vi "7HP_Channels.vi"(1 "Analysis Info cluster":T2[](array[typedef]) {"Sync Delay Time (s)" format="%.4f"; "Sd Error in Variance" format="%.2f"; "Skew_u" format="%.2f"; "% u'/U" format="%.2f"; "Sd Error in Mean" format="%.2f"; "Kurt_u" format="%.2f"; "u^4" format="%.2f"; "u^3" format="%.2f"; "U" format="%.2f"; "u^2" format="%.2f"}) -> (0 "7HP Info":T1(array[cluster]))   [LabVIEW 2017]
uses:
  Controls/Analysis_info_cluster.ctl
  Controls/Inst_type.ctl
  Controls/Instrument_Array.ctl
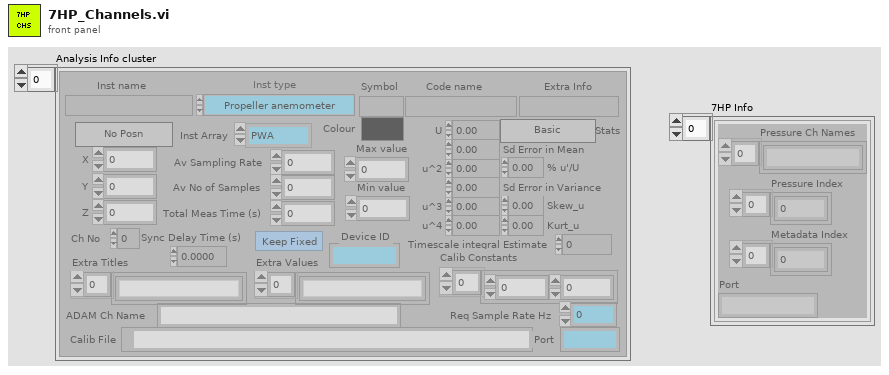
[diagram p1: front panel]
types:
  T1 = cluster{"Pressure Ch Names":string[], "Pressure Index":i32[], "Metadata Index":i32[], "Port":string}[]
  T2 = typedef "Analysis_info_cluster.ctl" = cluster{"Colour":u32, "Inst type":T3, "Inst name":string, "Symbol":string, "Code name":string, "Extra Info":string, "Inst Array":T4, "Extra Titles":string[], "Extra Values":string[], "U":dbl, "u^2":dbl, "u^3":dbl, "u^4":dbl, "Skew_u":dbl, "Kurt_u":dbl, "Sd Error in Mean":dbl, "% u'/U":dbl, "X":dbl, "Y":dbl, "Z":dbl, "Timescale integral Estimate":dbl, "Sd Error in Variance":dbl, "Calib File":path, "Calib Constants":dbl[], "Output Position":bool, "Full Stats":bool, "Av Sampling Rate":dbl, "Av No of Samples":dbl, "Total Meas Time (s)":dbl, "ADAM Ch Name":string, "Max value":dbl, "Min value":dbl, "Req Sample Rate Hz":dbl, "Sync Delay Time (s)":dbl, "Ch No":i16, "Device ID":string, "Use Latest Calib":bool, "Port":string}
  T3 = typedef "Inst_type.ctl" = enum16{"Propeller anemometer", "Raw voltage", "Pressure Transducer", "Pitot-static tube", "Preston tube", "Hot wire", "Cross wire 1", "Cross wire 2", "Generic Linear", "Generic Polynomial", "Generic BackPoly", "Fast FID", "Thermocouple", "Cold wire", "Pulsed Wire", "LDA Vel", "LDA Tran time", "LDA Arr time", "Microphone"}
  T4 = typedef "Instrument_Array.ctl" = enum16{"PWA", "LDA", "Analogue"}
  T5 = cluster{"Pressure Ch Names":string[], "Pressure Index":i32[], "Metadata Index":i32[], "Port":string}
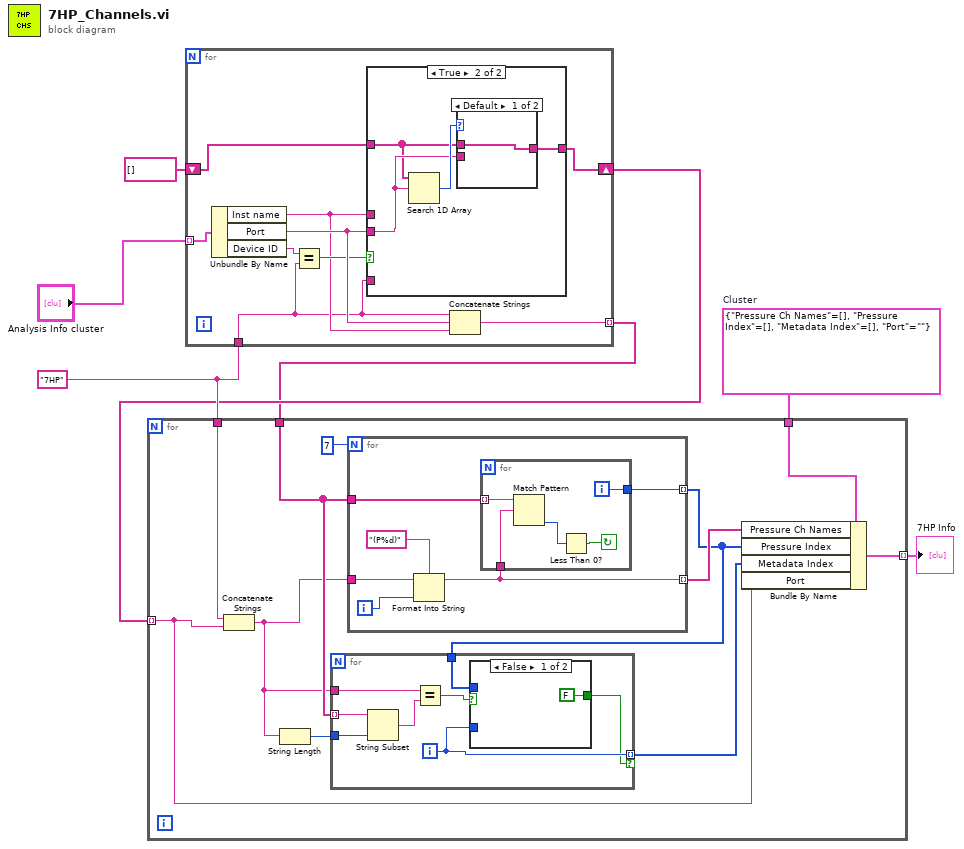
[diagram p0: block diagram]
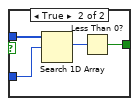
[diagram p2: hidden frame]
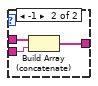
[diagram p4: hidden frame]
diagram:
  w2 = T5 {"Pressure Ch Names"=[], "Pressure Index"=[], "Metadata Index"=[], "Port"=""}  # Cluster
  w5 = "7HP" ("Device ID")
  n1 = for {
    tunnel: "Analysis Info cluster" -> [w11] mode=indexing
    shift-right: [w13] -> w4
    shift-left: string[] [] -> [w15]
    tunnel: [w9] -> w3 mode=indexing
    tunnel: w5 -> [w8]
    n2 = Unbundle By Name(w11) -> ("Inst name"=w10:string, "Port"=w14:string, "Device ID"=w16:string)
    n3 = Equal?(x=w16, y=w8) -> (x = y?=w12:bool)
    n4 = case shown="True" w12 {
      tunnel: w15 -> [w17 w18]
      tunnel: w14 -> [_ w19]
      tunnel: [w17 w20] -> w13
      tunnel: w8 -> [_ _]
      tunnel: w10 -> [_ _]
      frame False {
      }
      frame True {
        n5 = Search 1D Array(1D array=w18, element=w19) -> (index of element=w21:i32)  [unwired: 1 in]
        n6 = case shown="Default" w21 {
          tunnel: w18 -> [w22 w25]
          tunnel: w19 -> [_ w24]
          tunnel: [w22 w23] -> w20
          frame Default {
          }
          frame -1 {
            n7 = Build Array (concatenate)(w25, w24) -> (w23:string[])
          }
        }
      }
    }
    n8 = Concatenate Strings(w8, w14, w10) -> (w9:string)
  }
  n9 = for {
    tunnel: w5 -> [w36]
    tunnel: w4 -> [w32] mode=indexing
    tunnel: w3 -> [w30]
    tunnel: w2 -> [w34]
    tunnel: [w26] -> w1 mode=indexing
    n10 = Concatenate Strings(w36, w32) -> (w29:string)
    n11 = String Length(string=w29) -> (length=w31:i32)
    n12 = for {
      N: 7 -> [_]
      tunnel: w30 -> [w53]
      tunnel: [w52] -> w28 mode=indexing
      tunnel: w29 -> [w51]
      tunnel: [w50] -> w33 mode=indexing
      i -> [w55]
      n13 = Format Into String(format string="(P%d)", initial string=w51, w55) -> (resulting string=w50:string)  [unwired: 1 in, 1 out]
      n14 = for {
        tunnel: w53 -> [w56] mode=indexing
        tunnel: w50 -> [w60]
        tunnel: [w57] -> w52
        i -> [w57]
        stop <- w59 continue-if-true
        n15 = Match Pattern(string=w56, regular expression=w60) -> (offset past match=w58:i32)  [unwired: 1 in, 3 out]
        n16 = Less Than 0?(x=w58) -> (x < 0?=w59:bool)
      }
    }
    n17 = for {
      tunnel: w31 -> [w44]
      tunnel: w30 -> [w43] mode=indexing
      tunnel: w29 -> [w41]
      tunnel: w28 -> [w39]
      tunnel: [w38] -> w27 mode=indexing if=w37
      i -> [w38]
      n18 = String Subset(string=w43, length (rest)=w44) -> (substring=w42:string)  [unwired: 1 in]
      n19 = Equal?(x=w41, y=w42) -> (x = y?=w40:bool)
      n20 = case shown="False" w40 {
        tunnel: w39 -> [_ w49]
        tunnel: w38 -> [_ w48]
        tunnel: [FALSE w46] -> w37
        frame False {
        }
        frame True {
          n21 = Search 1D Array(1D array=w49, element=w48) -> (index of element=w47:i32)  [unwired: 1 in]
          n22 = Less Than 0?(x=w47) -> (x < 0?=w46:bool)
        }
      }
    }
    n23 = Bundle By Name(cluster=w34, "Pressure Ch Names"=w33, "Pressure Index"=w28, "Metadata Index"=w27, "Port"=w32) -> (w26:T5)
  }
  "7HP Info" <- w1
